vi "Get Class.vi"(8 "error in (no error)":errorcluster, 11 "MockTransceiver in":refnum<class "MockTransceiver.lvclass">) -> (0 "error out":errorcluster, 2 "class":string, 3 "MockTransceiver out":refnum<class "MockTransceiver.lvclass">)   [LabVIEW 2017, in "MockTransceiver.lvclass"]
uses:
  MockTransceiver.lvclass
  Engine/Classes/Transceiver/Transceiver.lvclass
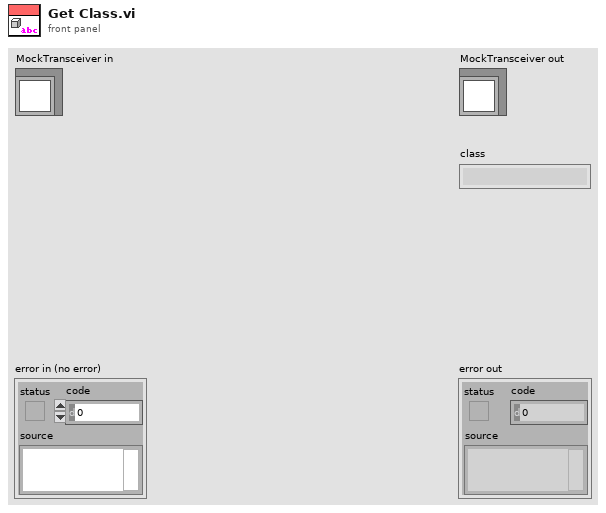
[diagram p1: front panel]
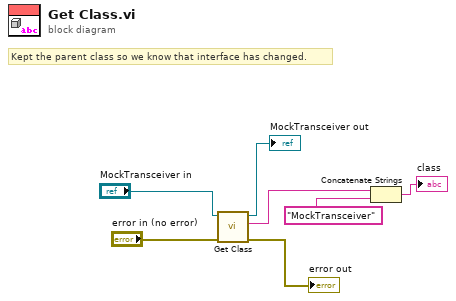
[diagram p0: block diagram]
diagram:
  # "Kept the parent class so we know that interface has changed."
  n1 = call-parent "Get Class.vi"("error in (no error)"="error in (no error)", "Transceiver in"="MockTransceiver in") -> ("error out"=→"error out":errorcluster, "class"=w3:string, "Transceiver out"=→"MockTransceiver out":refnum<class "MockTransceiver.lvclass">)  [unwired: 7 in]
  n2 = Concatenate Strings(w3, "MockTransceiver" ("string")) -> (→"class":string)
